vi "LVClass_WavefrontCorrectorSet WriteFile WavefrontCorrectorSetup.vi"(0 "WavefrontCorrectorSet in":refnum<class "WavefrontCorrectorSet.lvclass">, 11 "error in (no error)":errorcluster) -> (4 "WavefrontCorrectorSet out":refnum<class "WavefrontCorrectorSet.lvclass">, 15 "error out":errorcluster)   [LabVIEW 2020, in "WavefrontCorrectorSet.lvclass"]
uses:
  WavefrontCorrectorSet.lvclass
  CameraParametersSetup.ctl
  CameraParameters_Type.ctl
  Wavefront Corrector states.ctl
  Wavefront Corrector states - ONE.ctl
  WavefrontCorrectorSet.lvclass/WavefrontCorrectorSet.ctl
  Write to XML File(string).vi
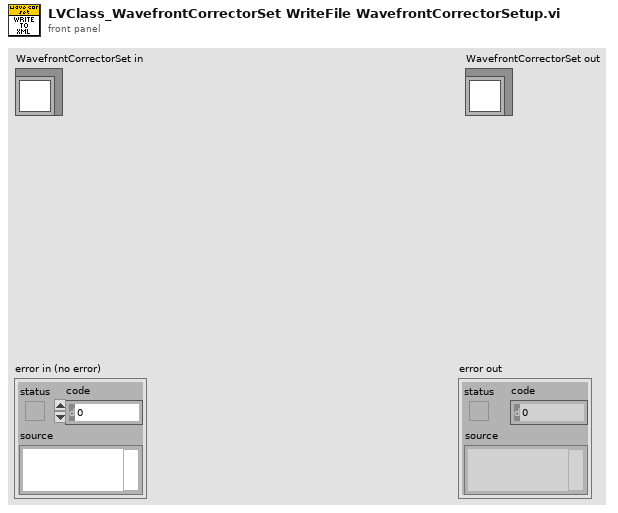
[diagram p1: front panel]
types:
  T1 = typedef "CameraParametersSetup.ctl" = cluster{"Name":string, "Type":T2, "Value":dbl, "BooleanValue":bool, "StringValue":string}
  T2 = typedef "CameraParameters_Type.ctl" = enum16{"Integer", "Real", "String", "Boolean"}
  T3 = typedef "Wavefront Corrector states.ctl" = cluster{"Sleep after command apply_ms":i32, "Wavefront Corrector State":T4[], "WavefrontCorrectorOffsetState":sgl[]}
  T4 = typedef "Wavefront Corrector states - ONE.ctl" = cluster{"Max":sgl, "Min":sgl, "Validity":enum16{"valid", "fixed", "invalid"}, "Fixed_Position":sgl}
  T5 = cluster{"AllWavefrontCorrectorParameters":T1[], "WavefrontCorrectorPreferences":T3}
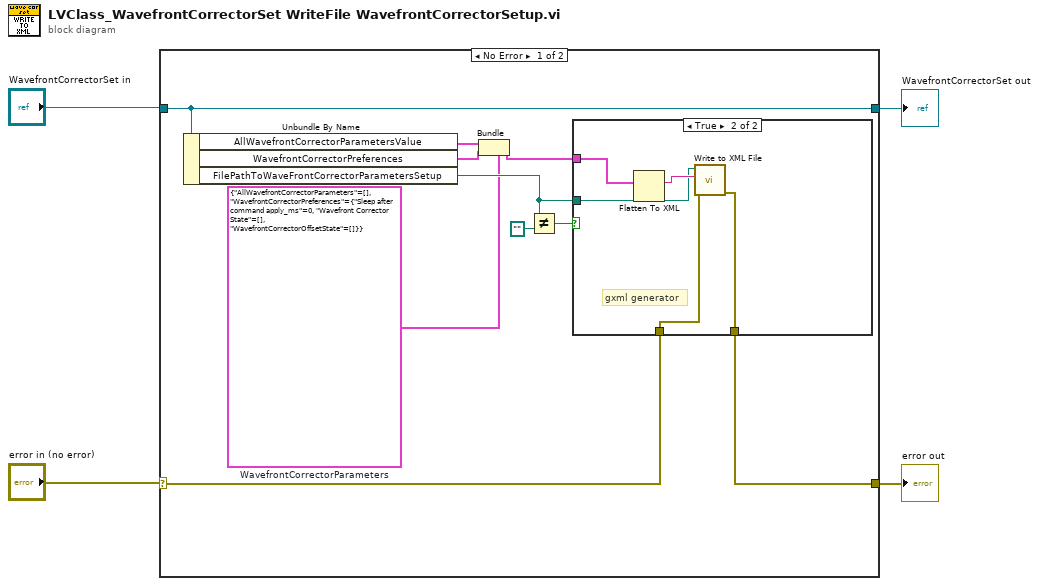
[diagram p0: block diagram]
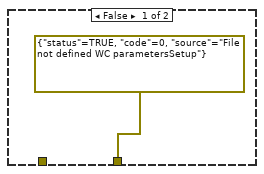
[diagram p2: hidden frame]
diagram:
  n1 = case shown="No Error" "error in (no error)" {
    selector: "error in (no error)" -> [w14 w22]
    tunnel: [w13 w22] -> w3
    tunnel: [w9 w21] -> w1
    tunnel: "WavefrontCorrectorSet in" -> [w9 w21]
    frame No Error {
      w7 = T5 {"AllWavefrontCorrectorParameters"=[], "WavefrontCorrectorPreferences"={"Sleep after command apply_ms"=0, "Wavefront Corrector State"=[], "WavefrontCorrectorOffsetState"=[]}}  # WavefrontCorrectorParameters
      n2 = Unbundle By Name(w9) -> ("AllWavefrontCorrectorParametersValue"=w8:T1[], "WavefrontCorrectorPreferences"=w6:T3, "FilePathToWaveFrontCorrectorParametersSetup"=w10:path)
      n3 = Bundle(cluster=w7, "AllWavefrontCorrectorParameters"=w8, "WavefrontCorrectorPreferences"=w6) -> (w5:T5)
      n4 = Not Equal?(x=w10, y=path "") -> (x != y?=w11:bool)
      n5 = case shown="True" w11 {
        tunnel: w5 -> [_ w19]
        tunnel: w10 -> [_ w18]
        tunnel: w14 -> [_ w16]
        tunnel: [errorcluster {"status"=TRUE, "code"=0, "source"="File not defined WC parametersSetup"} ("error out") w17] -> w13
        frame False {
        }
        frame True {
          # "gxml generator"
          n6 = Flatten To XML(6:w19) -> (2:w20:string)
          n7 = call-poly "Write to XML File.vi"("error in (no error)"=w16, "XML Input"=w20, "XML File Path"=w18) -> ("error out"=w17:errorcluster)  [unwired: 6 in, 2 out]
        }
      }
    }
    frame Error {
    }
  }
  "error out" <- w3
  "WavefrontCorrectorSet out" <- w1
